vi "Config Dev Bounds.vi"(6 "Lower Loss (-0.1 jpF)":dbl=-0.1 min=-1900.0 max=19000.0 format="%#_6f", 7 "Upper Capacitance (101 pF)":dbl=101.0 min=-165000.0 max=1650000.0 format="%#_6f", 8 "error in":errorcluster, 9 "Lower Capacitance (99 pF)":dbl=99.0 min=-165000.0 max=1650000.0 format="%#_6f", 10 "Upper Loss (0.1 jpF)":dbl=1900.0 min=-1900.0 max=19000.0 format="%#_6f", 11 "VISA resource name":refnum<visa-resource-name>) -> (0 "error out":errorcluster, 3 "VISA resource name out":refnum<visa-resource-name>)   [LabVIEW 2014, in "Andeen-Hagerling 2700.lvlib"]
uses:
  Andeen-Hagerling 2700.lvlib
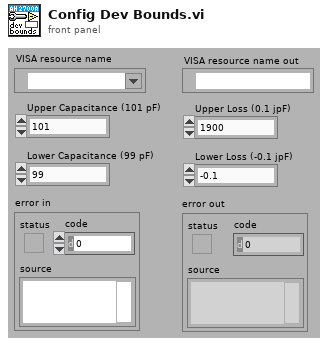
[diagram p1: front panel]
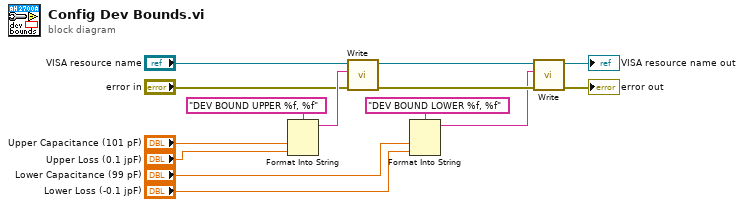
[diagram p0: block diagram]
diagram:
  n1 = Format Into String(format string="DEV BOUND UPPER %f, %f", "Upper Capacitance (101 pF)", "Upper Loss (0.1 jpF)") -> (resulting string=w13:string)  [unwired: 2 in, 1 out]
  n2 = call "Write.vi"("error in"="error in", "command"=w13, "VISA resource name"="VISA resource name") -> ("error out"=w11:errorcluster, "VISA resource name out"=w12:refnum<visa-resource-name>)  [unwired: 7 in]
  n3 = Format Into String(format string="DEV BOUND LOWER %f, %f", "Lower Capacitance (99 pF)", "Lower Loss (-0.1 jpF)") -> (resulting string=w10:string)  [unwired: 2 in, 1 out]
  n4 = call "Write.vi"("error in"=w11, "command"=w10, "VISA resource name"=w12) -> ("error out"=→"error out":errorcluster, "VISA resource name out"=→"VISA resource name out":refnum<visa-resource-name>)  [unwired: 7 in]
